vi "Serial_Port_Write.vi"(1 "Write String":string, 2 "dup VISA resource name":refnum<visa-resource-name>) -> (0 "error out":errorcluster)   [LabVIEW 2011]
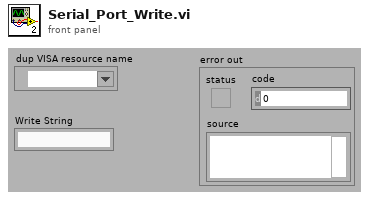
[diagram p1: front panel]
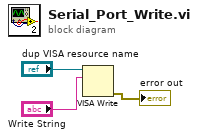
[diagram p0: block diagram]
diagram:
  n1 = VISA Write(VISA resource name="dup VISA resource name", write buffer="Write String") -> (error out=→"error out":errorcluster)  [unwired: 1 in, 2 out]
